vi "2100_Trim_Meas_PI1.vi"(7 "Delay Time (s)":dbl=0.001 format="%#_13p", 10 "Pins":string[](array[string])=["PI0"], 11 "Semiconductor Module Context":T1) -> (0 "error out":errorcluster, 3 "PI_1_Meas":dbl format="%#_6p")   [LabVIEW 2013]
uses:
  <vilib>/NI_TestStand_SemiconductorModule/NI_TestStand_Semiconductor_Module.lvlibp/PinMap/General/SemiconductorModuleContext.ctl
  <vilib>/NI_TestStand_SemiconductorModule/NI_TestStand_Semiconductor_Module.lvlibp/PinMap/DC Power/PinsToNIDCPowerSessions.vi
  <vilib>/NI_TestStand_SemiconductorModule/NI_TestStand_Semiconductor_Module.lvlibp
panel:
  in  "error in":errorcluster
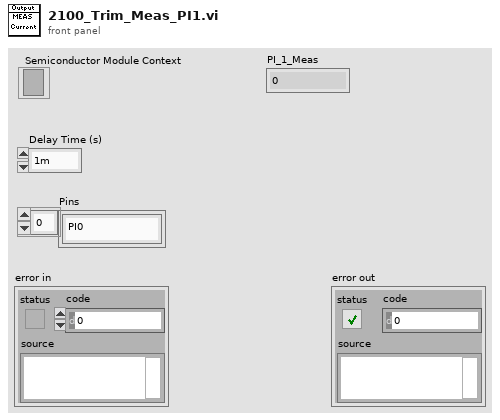
[diagram p1: front panel]
types:
  T1 = typedef "NI_TestStand_Semiconductor_Module.lvlibp/SemiconductorModuleContext.ctl" = refnum<k7>
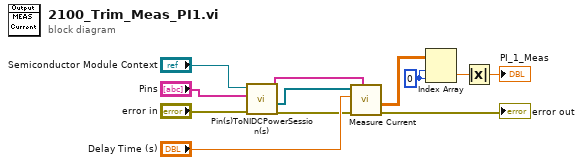
[diagram p0: block diagram]
diagram:
  w3 = 0 ("disabled index (col)")
  n1 = call-poly <vilib>:"Pin(s)ToNIDCPowerSession(s).vi"("error in (no error)"="error in", "Pins"="Pins", "Semiconductor Module Context"="Semiconductor Module Context") -> ("error out"=w9:errorcluster, "Instrument Sessions"=w8:refnum<k15>[], "Channel Lists"=w11:string[])  [unwired: 4 in, 2 out]
  n2 = call "Measure Current.vi"("Channel Lists"=w11, "error in (no error)"=w9, "Delay Time (s)"="Delay Time (s)", "DCPower Sessions In"=w8) -> ("error out"=→"error out":errorcluster, "current measurements"=w4:dbl[][])  [unwired: 5 in, 1 out]
  n3 = Index Array(array=w4, index (row)=w3, index (col)=w3) -> (element=w2:dbl)
  n4 = Absolute Value(x=w2) -> (abs(x)=→"PI_1_Meas":dbl)
